vi "Lock Front Panel.vi"(8 "error in (no error)":errorcluster, 10 "Lock?":bool, 11 "N5745A in":refnum<class "5745A.lvclass">) -> (0 "error out":errorcluster, 3 "N5745A out":refnum<class "5745A.lvclass">)   [LabVIEW 2018, in "5745A.lvlib" / "5745A.lvclass"]
doc: "This VI allows the program to lock out front panel controls or unlock them."
uses:
  5745A.lvclass
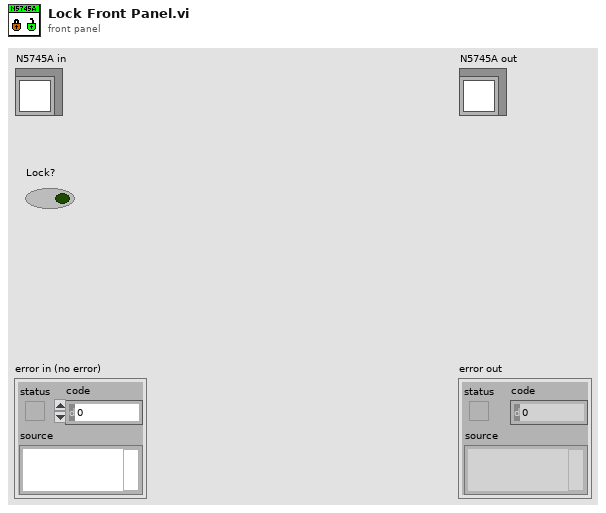
[diagram p1: front panel]
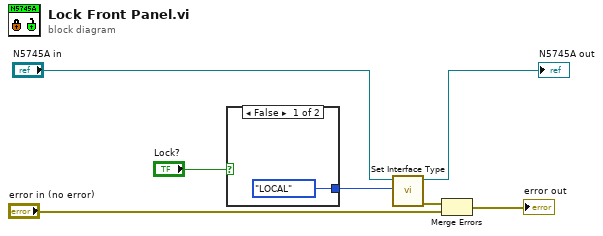
[diagram p0: block diagram]
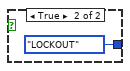
[diagram p2: hidden frame]
diagram:
  n1 = case shown="False" "Lock?" {
    tunnel: [enum16{"LOCAL", "REMOTE", "LOCKOUT"}."LOCAL" ("Mode") enum16{"LOCAL", "REMOTE", "LOCKOUT"}."LOCKOUT" ("Mode")] -> w3
    frame False {
    }
    frame True {
    }
  }
  n2 = call "Set Interface Type.vi"("Mode"=w3, "N5745A in"="N5745A in") -> ("error out"=w5:errorcluster, "N5745A out"=→"N5745A out":refnum<class "5745A.lvclass">)  [unwired: 8 in]
  n3 = Merge Errors(w5, "error in (no error)") -> (→"error out":errorcluster)
